vi "setBK1823ACounter.vi"(8 "error in (no error)":errorcluster, 10 "Hardware:FrequencyCounters:BK1823ACounter.lvclass":refnum<class "BK1823ACounter.lvclass">, 11 "frequencyCounterController.lvclass in":refnum<class "frequencyCounterController.lvclass">) -> (0 "error out":errorcluster, 3 "frequencyCounterController.lvclass out":refnum<class "frequencyCounterController.lvclass">)   [LabVIEW 2011, in "Hardware.lvlib" / "frequencyCounters.lvlib" / "frequencyCounterController.lvclass"]
uses:
  frequencyCounterController.lvclass
  BK1823ACounter/BK1823ACounter.lvclass
  frequencyCounterController.lvclass/frequencyCounterController.ctl
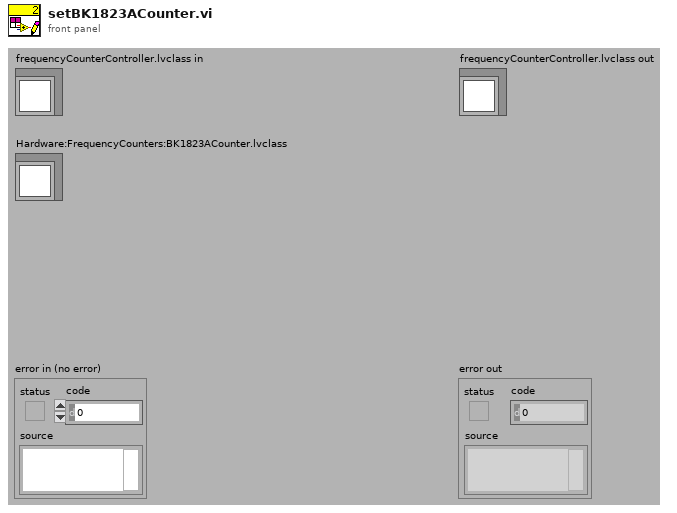
[diagram p1: front panel]
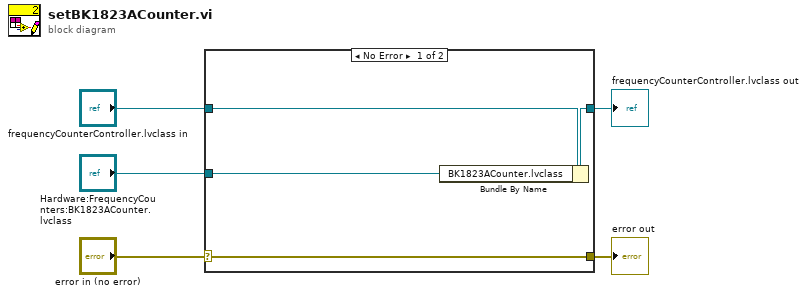
[diagram p0: block diagram]
diagram:
  n1 = case shown="No Error" "error in (no error)" {
    selector: "error in (no error)" -> [w9 w10]
    tunnel: [w9 w10] -> w4
    tunnel: [w7 w11] -> w2
    tunnel: "frequencyCounterController.lvclass in" -> [w8 w11]
    tunnel: "Hardware:FrequencyCounters:BK1823ACounter.lvclass" -> [w6 _]
    frame No Error {
      n2 = Bundle By Name(cluster=w8, "BK1823ACounter.lvclass"=w6) -> (w7:refnum<class "frequencyCounterController.lvclass">)
    }
    frame Error {
    }
  }
  "error out" <- w4
  "frequencyCounterController.lvclass out" <- w2
